vi "Retrieve.vi"(7 "Description":string, 8 "Command Info In":T3) -> (0 "Command Info":T3, 3 "SubSystem Data":T1)   [LabVIEW 2015]
uses:
  <vilib>/Rock Robotics/WPI/Framework/Command Status Info.ctl
  <vilib>/Rock Robotics/WPI/Framework/Completion Status.ctl
  <vilib>/Rock Robotics/WPI/Framework/Completion Notifier.ctl
  Implementation/LowShooter Setpoints.ctl
  Implementation/LowShooter Operations.ctl
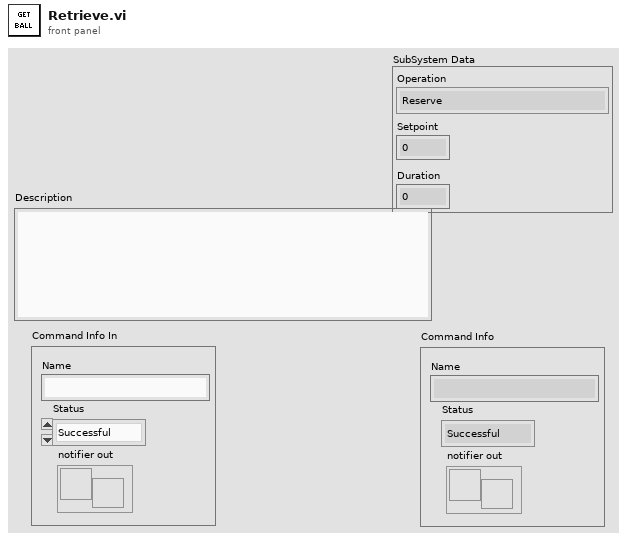
[diagram p1: front panel]
types:
  T1 = typedef "LowShooter Setpoints.ctl" = cluster{"Operation":T2, "Setpoint":dbl, "Duration":dbl}
  T2 = typedef "LowShooter Operations.ctl" = enum16{"Reserve", "Read Current", "Immediate", "Shoot", "Retrieve", "Move Arm Down"}
  T3 = typedef "Command Status Info.ctl" = cluster{"Name":string, "Status":T4, "notifier out":T5}
  T4 = typedef "Completion Status.ctl" = enum16{"Successful", "Aborted", "Incomplete"}
  T5 = typedef "Completion Notifier.ctl" = refnum<notifier>
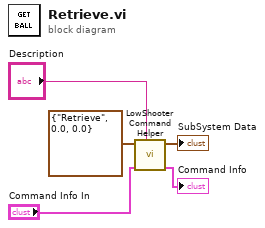
[diagram p0: block diagram]
diagram:
  n1 = call "LowShooter Command Helper.vi"("Description"="Description", "Command Info In"="Command Info In", "SubSystem Data"=T1 {"Operation"=enum."Retrieve", "Setpoint"=0.0, "Duration"=0.0}) -> ("Command Info Out"=→"Command Info":T3, "SubSystem Data"=→"SubSystem Data":T1)  [unwired: 7 in]
